vi "Read Pass Fail.vi"(8 "error in (no error)":errorcluster, 11 "Results in":refnum<class "Results.lvclass">) -> (0 "error out":errorcluster, 2 "Pass Fail":bool, 3 "Results out":refnum<class "Results.lvclass">)   [LabVIEW 2016, in "TestStand API.lvlib"]
uses:
  TestStand API.lvlib
  MAL-Framework/user.lib/Common Components/Results/Results.lvclass
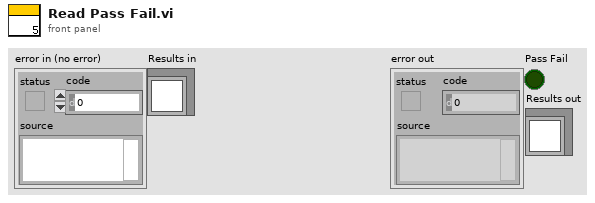
[diagram p1: front panel]
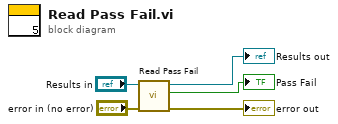
[diagram p0: block diagram]
diagram:
  n1 = call "Read Pass Fail.vi"("error in (no error)"="error in (no error)", "Results in"="Results in") -> ("error out"=→"error out":errorcluster, "Pass Fail"=→"Pass Fail":bool, "Results out"=→"Results out":refnum<class "Results.lvclass">)  [unwired: 7 in]
